vi "FormatDurationText.vi"(10 "Duration [s]":dbl) -> (2 "String":string)   [LabVIEW 2019, in "ResultTree.lvclass"]
doc: "Returns the text representation for a given duration. The duration is defined in seconds."
uses:
  ResultTree.lvclass
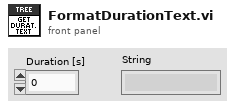
[diagram p1: front panel]
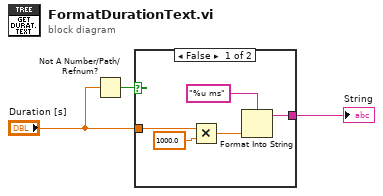
[diagram p0: block diagram]
diagram:
  n1 = Not A Number/Path/Refnum?(number/path/refnum="Duration [s]") -> (NaN/Path/Refnum?=w2:bool)
  n2 = case shown="False" w2 {
    tunnel: "Duration [s]" -> [w8 _]
    tunnel: [w4 _] -> w3
    frame False {
      n3 = Multiply(x=w8, y=1000.0) -> (x*y=w6:dbl)
      n4 = Format Into String(format string="%u ms", w6) -> (resulting string=w4:string)  [unwired: 2 in, 1 out]
    }
    frame True {
    }
  }
  "String" <- w3
